vi "Read.vi"(11 "GroupsAbstractValue in":refnum<class "GroupsAbstractValue.lvclass">) -> (2 "Groups":refnum<class "Group.lvclass">[](array[class]))   [LabVIEW 2020, in "Vecto.lvlib" / "GroupsAbstractValue.lvclass"]
uses:
  GroupsAbstractValue.lvclass
  Group/Group.lvclass
  GroupsAbstractValue.lvclass/GroupsAbstractValue.ctl
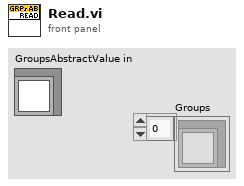
[diagram p1: front panel]
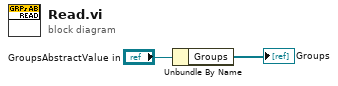
[diagram p0: block diagram]
diagram:
  n1 = Unbundle By Name("GroupsAbstractValue in") -> ("Groups"=→"Groups":refnum<class "Group.lvclass">[])
